vi "Unit Test.vi"() -> ()   [LabVIEW 2017]
uses:
  builds/Flash Utility.lvlibp/Flash Utility.lvclass
panel:
  in  "Erase":bool
  in  "stop":bool
  out "User Message":string
  out "Success":bool
  in  "Validate":bool
  in  "Flash":bool
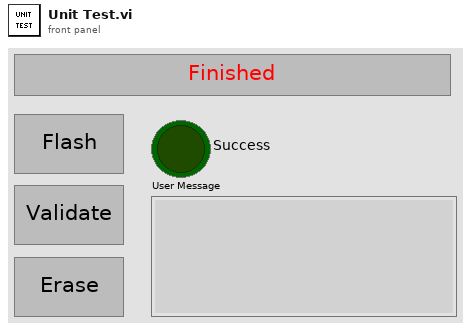
[diagram p1: front panel]
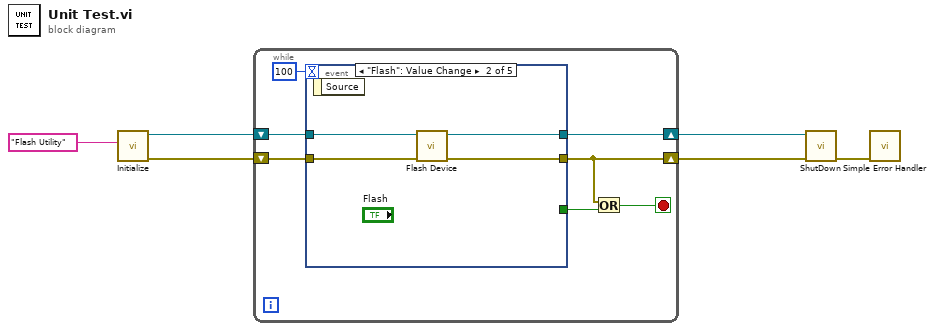
[diagram p0: block diagram]
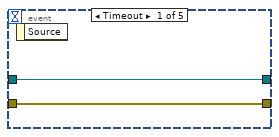
[diagram p2: hidden frame]
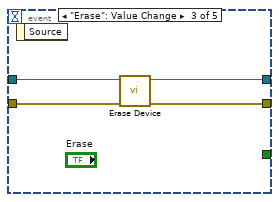
[diagram p3: hidden frame]
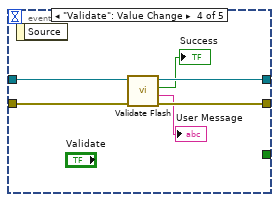
[diagram p4: hidden frame]
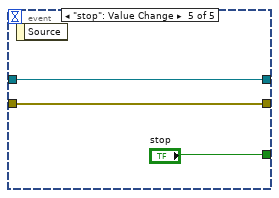
[diagram p5: hidden frame]
diagram:
  n1 = call "Initialize.vi"("Device"="Flash Utility") -> ("error out"=w4:errorcluster, "Flash Utility out"=w6:refnum<class "Flash Utility.lvclass">)  [unwired: 9 in]
  n2 = while {
    shift-right: [w12] -> w5
    shift-left: w6 -> [w13]
    shift-right: [w8] -> w2
    shift-left: w4 -> [w11]
    stop <- w7 stop-if-true
    n3 = event shown="[1] \"Flash\": Value Change" {
      selector: _ -> [_ _ _ _ _]
      dyn-events: _ -> [_ _ _ _ _]
      timeout: 100 -> [_ _ _ _ _]
      tunnel: w13 -> [w15 w18 w23 w29 w32]
      tunnel: [w15 w17 w22 w28 w32] -> w12
      tunnel: w11 -> [w14 w19 w21 w27 w31]
      tunnel: [w14 w16 w20 w26 w31] -> w8
      tunnel: [_ _ _ _ "stop"] -> w9
      event Timeout {
        n4 = event-data() -> ()  [unwired: 1 in, 1 out]
      }
      event "Flash": Value Change {
        n5 = event-data() -> ()  [unwired: 1 in, 1 out]
        n6 = call-dynamic "Flash Device.vi"("error in (no error)"=w19, "Flash Utility in"=w18) -> ("error out"=w16:errorcluster, "Flash Utility out"=w17:refnum<class "Flash Utility.lvclass">)  [unwired: 8 in]
      }
      event "Erase": Value Change {
        n7 = event-data() -> ()  [unwired: 1 in, 1 out]
        n8 = call-dynamic "Erase Device.vi"("error in (no error)"=w21, "Flash Utility in"=w23) -> ("error out"=w20:errorcluster, "Flash Utility out"=w22:refnum<class "Flash Utility.lvclass">)  [unwired: 8 in]
      }
      event "Validate": Value Change {
        n9 = event-data() -> ()  [unwired: 1 in, 1 out]
        n10 = call-dynamic "Validate Flash.vi"("error in (no error)"=w27, "Flash Utility in"=w29) -> ("error out"=w26:errorcluster, "Failure Message"=→"User Message":string, "Success?"=→"Success":bool, "Flash Utility out"=w28:refnum<class "Flash Utility.lvclass">)  [unwired: 6 in]
      }
      event "stop": Value Change {
        n11 = event-data() -> ()  [unwired: 1 in, 1 out]
      }
    }
    n12 = Or(x=w8, y=w9) -> (x .or. y?=w7:bool)
  }
  n13 = call "ShutDown.vi"("error in (no error)"=w2, "Flash Utility in"=w5) -> ("error out"=w1:errorcluster)  [unwired: 8 in, 1 out]
  n14 = call <vilib>:"Simple Error Handler.vi"("error in (no error)"=w1) -> ()  [unwired: 4 in, 5 out]
